vi "Syncronous detector.vi"(7 "Initialize?":bool, 8 "error in (no error)":errorcluster, 10 "data":waveform(dbl)[](array[waveform]), 11 "Lock-in settings":T1={"Sine Frequency, Hz"=0.0, "Time constant, s"=0.12500000000000006, "Low-pass filter"=enum."No filtering", "Output representation"=enum."Real/Imaginary", "Phases, deg"=[], "Low-pass filter Order"=1, "Decimating factor"=1, "Samples to Read"=10000, "Post-filter decimation"=1, "Blocks to average"=1, "Trig delay, points"=0, "Harmonics per channel"=[], "Amplitude scale"=enum."RMS"} {"Time constant, s" format="%.1e"}) -> (0 "error out":errorcluster, 2 "signal(s) out":waveform(dbl)[](array[waveform]), 3 "Lock-in settings out":T1={"Sine Frequency, Hz"=0.0, "Time constant, s"=0.12500000000000006, "Low-pass filter"=enum."No filtering", "Output representation"=enum."Real/Imaginary", "Phases, deg"=[], "Low-pass filter Order"=1, "Decimating factor"=1, "Samples to Read"=10000, "Post-filter decimation"=1, "Blocks to average"=1, "Trig delay, points"=0, "Harmonics per channel"=[], "Amplitude scale"=enum."RMS"} {"Time constant, s" format="%.1e"})   [LabVIEW 2015]
uses:
  Controls/Lockin Settings.ctl
  Controls/Harmonics per channel.ctl
  <vilib>/Analysis/2dsp.llb/Decimate (single shot, DBL).vi
  <vilib>/Analysis/NI_AALPro.lvlib
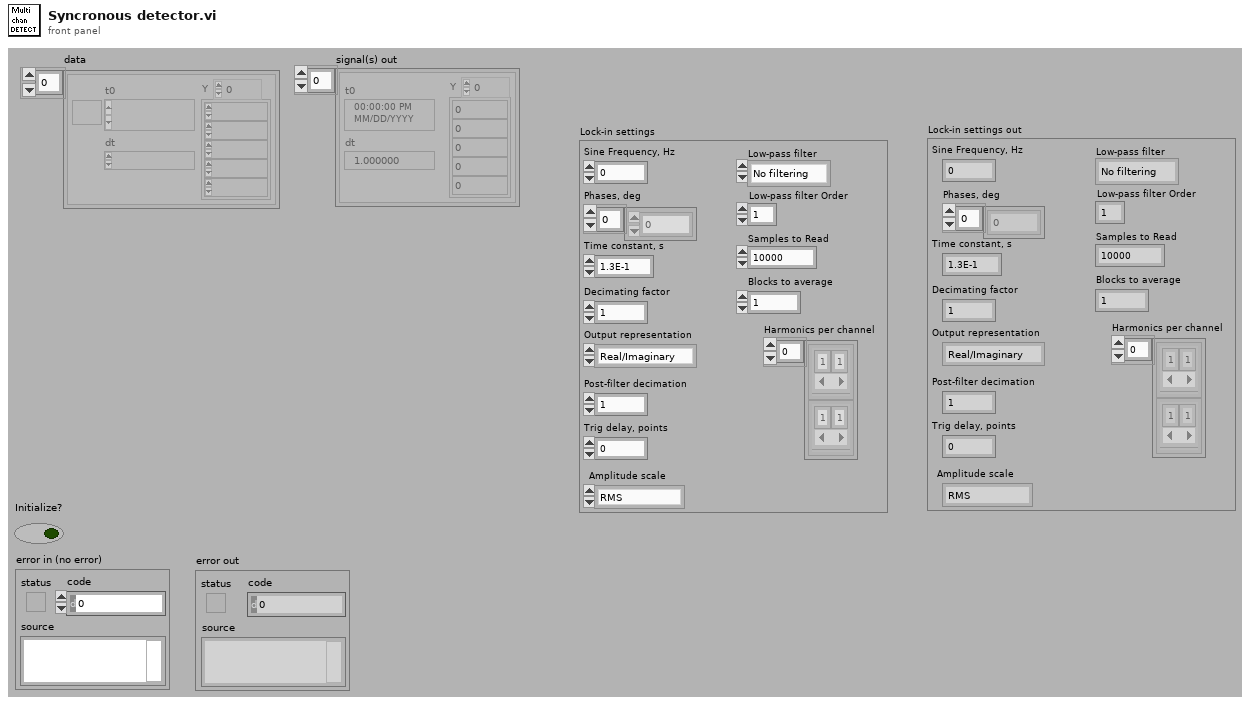
[diagram p1: front panel]
types:
  T1 = typedef "Lockin Settings.ctl" = cluster{"Sine Frequency, Hz":dbl, "Time constant, s":dbl, "Low-pass filter":enum16{"No filtering", "Butterworth", "Bessel"}, "Output representation":enum16{"Real/Imaginary", "Polar"}, "Phases, deg":dbl[], "Low-pass filter Order":i32, "Decimating factor":i32, "Samples to Read":i32, "Post-filter decimation":i32, "Blocks to average":i32, "Trig delay, points":i32, "Harmonics per channel":T2, "Amplitude scale":enum16{"Amplitude", "RMS", "Peak-to-Peak"}}
  T2 = typedef "Harmonics per channel.ctl" = cluster{"Harmonics":i32[]}[]
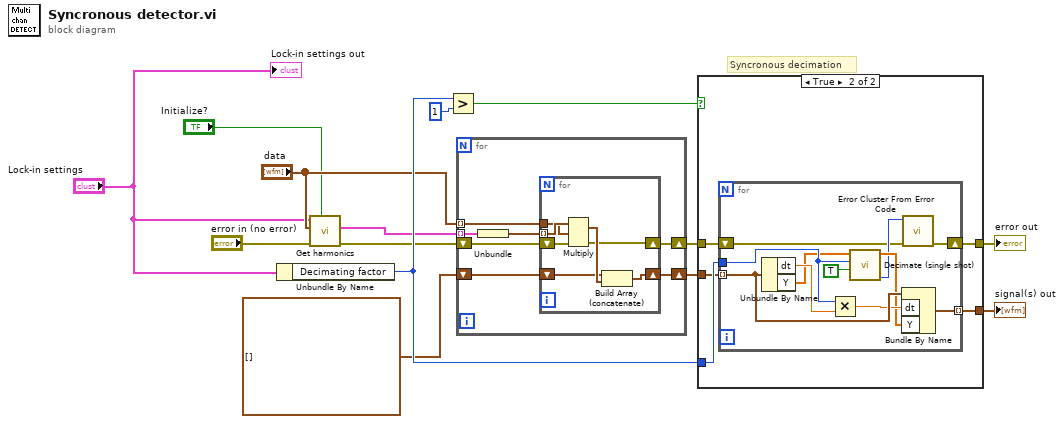
[diagram p0: block diagram]
diagram:
  # "Syncronous decimation"
  n1 = Unbundle By Name("Lock-in settings") -> ("Decimating factor"=w12:i32)
  n2 = call "Get harmonics.vi"("Initialize?"="Initialize?", "error in (no error)"="error in (no error)", "data"="data", "Lock-in settings"="Lock-in settings") -> ("error out"=w5:errorcluster, "Harmonics"=w8:cluster{waveform(dbl)[]}[])  [unwired: 5 in, 1 out]
  n3 = Greater?(x=w12, y=1) -> (0:w13:bool)
  n4 = for {
    tunnel: w8 -> [w21] mode=indexing
    shift-right: [w18] -> w6
    shift-left: waveform(dbl)[] [] -> [w19]
    shift-right: [w16] -> w4
    shift-left: w5 -> [w17]
    tunnel: "data" -> [w15] mode=indexing
    n5 = Unbundle(w21) -> (w20:waveform(dbl)[])
    n6 = for {
      tunnel: w20 -> [w23] mode=indexing
      shift-right: [w26] -> w18
      shift-left: w19 -> [w27]
      shift-right: [w24] -> w16
      shift-left: w17 -> [w25]
      tunnel: w15 -> [w22]
      n7 = Multiply(1:w22, 2:w23, 4:w25) -> (0:w28:waveform(dbl), 3:w24:errorcluster)
      n8 = Build Array (concatenate)(w27, w28) -> (w26:waveform(dbl)[])
    }
  }
  n9 = case shown="True" w13 {
    tunnel: w12 -> [_ w35]
    tunnel: w6 -> [w30 w34]
    tunnel: [w30 w33] -> w10
    tunnel: w4 -> [w29 w32]
    tunnel: [w29 w31] -> w11
    frame False {
    }
    frame True {
      n10 = for {
        tunnel: w35 -> [w43]
        tunnel: w34 -> [w45] mode=indexing
        tunnel: [w39] -> w33 mode=indexing
        shift-right: [w36] -> w31
        shift-left: w32 -> [w37]
        n11 = Unbundle By Name(w45) -> ("dt"=w44:dbl, "Y"=w40:dbl[])
        n12 = Multiply(x=w43, y=w44) -> (x*y=w42:dbl)
        n13 = call-poly <vilib>:"Decimate (single shot).vi"("averaging"=TRUE, "decimating factor"=w43, "X"=w40) -> ("error"=w38:i32, "Decimated Array"=w41:dbl[])  [unwired: 7 out]
        n14 = Bundle By Name(cluster=w45, "dt"=w42, "Y"=w41) -> (w39:waveform(dbl))
        n15 = call <vilib>:"Error Cluster From Error Code.vi"("error in (no error)"=w37, "error code (0)"=w38) -> ("error out"=w36:errorcluster)  [unwired: 1 in, 6 out]
      }
    }
  }
  "signal(s) out" <- w10
  "error out" <- w11
  "Lock-in settings out" <- "Lock-in settings"
